vi "WinCI File Properties.vi"(8 "error in (no error)":errorcluster, 10 "filename":path, 11 "source control reference in":T1) -> (0 "error out":errorcluster, 2 "status message":string, 3 "source control reference out":T1, 5 "file changed?":bool)   [LabVIEW 2017, in "NI_SCC_WinCI.lvlib"]
uses:
  <vilib>/SourceControl/Providers/WinCI/NI_SCC_WinCI.lvlib
  <vilib>/SourceControl/sccapi/SCCAPI Refnum.ctl
  <vilib>/SourceControl/support/SCCSup Message Strings GLBL.vi
  <vilib>/SourceControl/sccapi/NI_SCC.lvlib
panel:
  out "result":i32
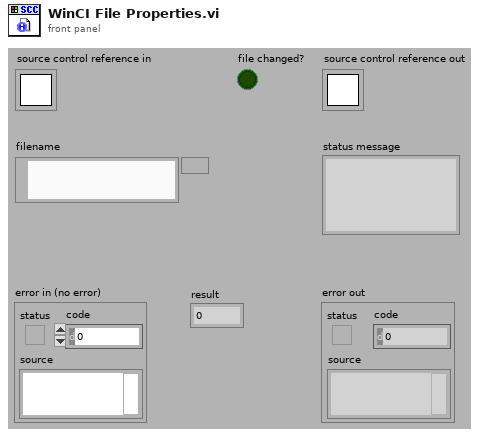
[diagram p1: front panel]
types:
  T1 = typedef "NI_SCC.lvlib/SCCAPI Refnum.ctl" = refnum<k1>
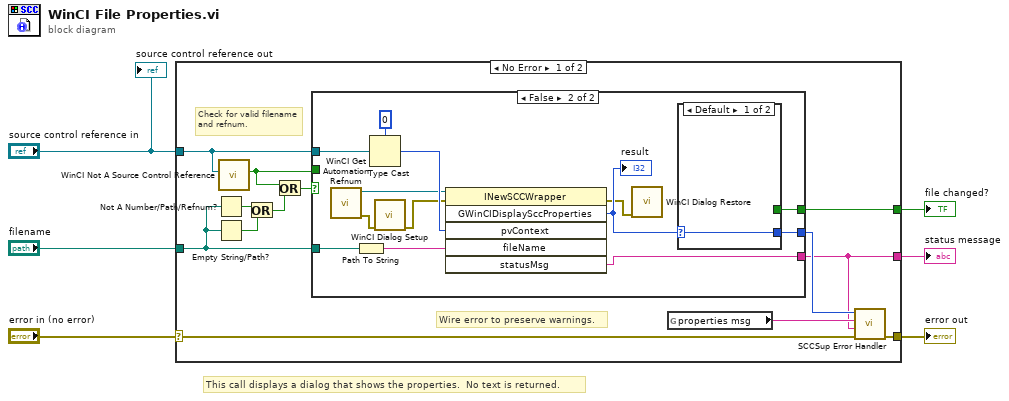
[diagram p0: block diagram]
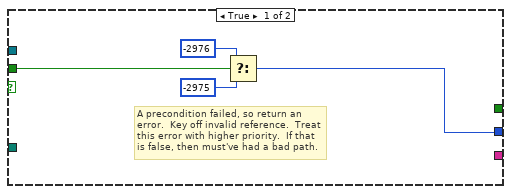
[diagram p2: hidden frame]
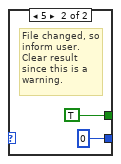
[diagram p3: hidden frame]
diagram:
  # "This call displays a dialog that shows the properties.  No text is returned."
  n1 = case shown="No Error" "error in (no error)" {
    selector: "error in (no error)" -> [w10 w40]
    tunnel: [w19 w40] -> w5
    tunnel: "source control reference in" -> [w7 _]
    tunnel: [w16 _] -> w3
    tunnel: "filename" -> [w12 _]
    tunnel: [w9 _] -> w1
    frame No Error {
      # "Wire error to preserve warnings."
      # "Check for valid filename and refnum."
      n2 = Not A Number/Path/Refnum?(number/path/refnum=w12) -> (NaN/Path/Refnum?=w13:bool)
      n3 = Empty String/Path?(string/path=w12) -> (empty?=w14:bool)
      n4 = call <vilib>:"WinCI Not A Source Control Reference.vi"("source control reference in"=w7) -> ("not a source control reference?"=w8:bool)  [unwired: 1 in, 9 out]
      n5 = Or(x=w13, y=w14) -> (x .or. y?=w15:bool)
      n6 = Or(x=w8, y=w15) -> (x .or. y?=w11:bool)
      n7 = case shown="False" w11 {
        tunnel: w7 -> [_ w36]
        tunnel: [_ w29] -> w16
        tunnel: w12 -> [_ w34]
        tunnel: [w20 w33] -> w18
        tunnel: w8 -> [w21 _]
        tunnel: [_ w32] -> w9
        frame True {
          # "A precondition failed, so return an error.  Key off invalid reference.  Treat this error with higher priority.  If that is false, then must've had a bad path."
          n8 = Select(t=-2976 ("result"), s=w21, f=-2975 ("result")) -> (s? t:f=w20:i32)
        }
        frame False {
          n9 = call <vilib>:"WinCI Get Automation Refnum.vi"() -> ("error out"=w26:errorcluster, "automation refnum"=w27:refnum<k7>)  [unwired: 10 out]
          n10 = Path To String(path=w34) -> (string=w30:string)
          n11 = Type Cast(type=u32 0, x=w36) -> (*(type *) &x=w31:u32)
          n12 = call <vilib>:"WinCI Dialog Setup.vi"("error in"=w26) -> ("error out"=w25:errorcluster)  [unwired: 10 out]
          n13 = invoke class="INewSCCWrapper" method="GWinCIDisplaySccProperties"(reference=w27, error in=w25, "pvContext"=w31, "fileName"=w30) -> (error out=w24:errorcluster, "GWinCIDisplaySccProperties"=w28:i32, "statusMsg"=w29:string)  [unwired: 2 in, 3 out]
          "result" <- w28
          n14 = call <vilib>:"WinCI Dialog Restore.vi"("error in"=w24) -> ()  [unwired: 11 out]
          n15 = case shown="Default" w28 {
            selector: w28 -> [w37 _]
            tunnel: [w37 0 ("result")] -> w33
            tunnel: [_ TRUE] -> w32
            frame Default {
            }
            frame 5 {
              # "File changed, so inform user.  Clear result since this is a warning."
            }
          }
        }
      }
      n16 = global read "SCCSup Message Strings GLBL.vi" "properties msg"() -> (w17:string)
      n17 = call <vilib>:"SCCSup Error Handler.vi"("error in (no error)"=w10, "additional message"=w16, "operation message"=w17, "scc error code"=w18) -> ("error out"=w19:errorcluster)  [unwired: 7 out]
    }
    frame Error {
    }
  }
  "error out" <- w5
  "status message" <- w3
  "file changed?" <- w1
  "source control reference out" <- "source control reference in"
